vi "VI Tree.vi"   [LabVIEW 2020, in "Rohde&Schwarz CMXP GPRF.lvlib"]
doc: "This is the instrument driver for the R&S CMXP Radiocommunication Analyzer GPRF.\n\nThe VI Tree displays all the user-callable VIs of the instrument driver in an organized \ntable.\n\nFor detailed driver information including modification history, refer to the <B>rscmxpgprf.chm </B> file."
uses:
  <instrlib>/Rohde&Schwarz CMXP GPRF/Rohde&Schwarz CMXP GPRF.lvlib
panel:
  # "rsCmxpGprf"
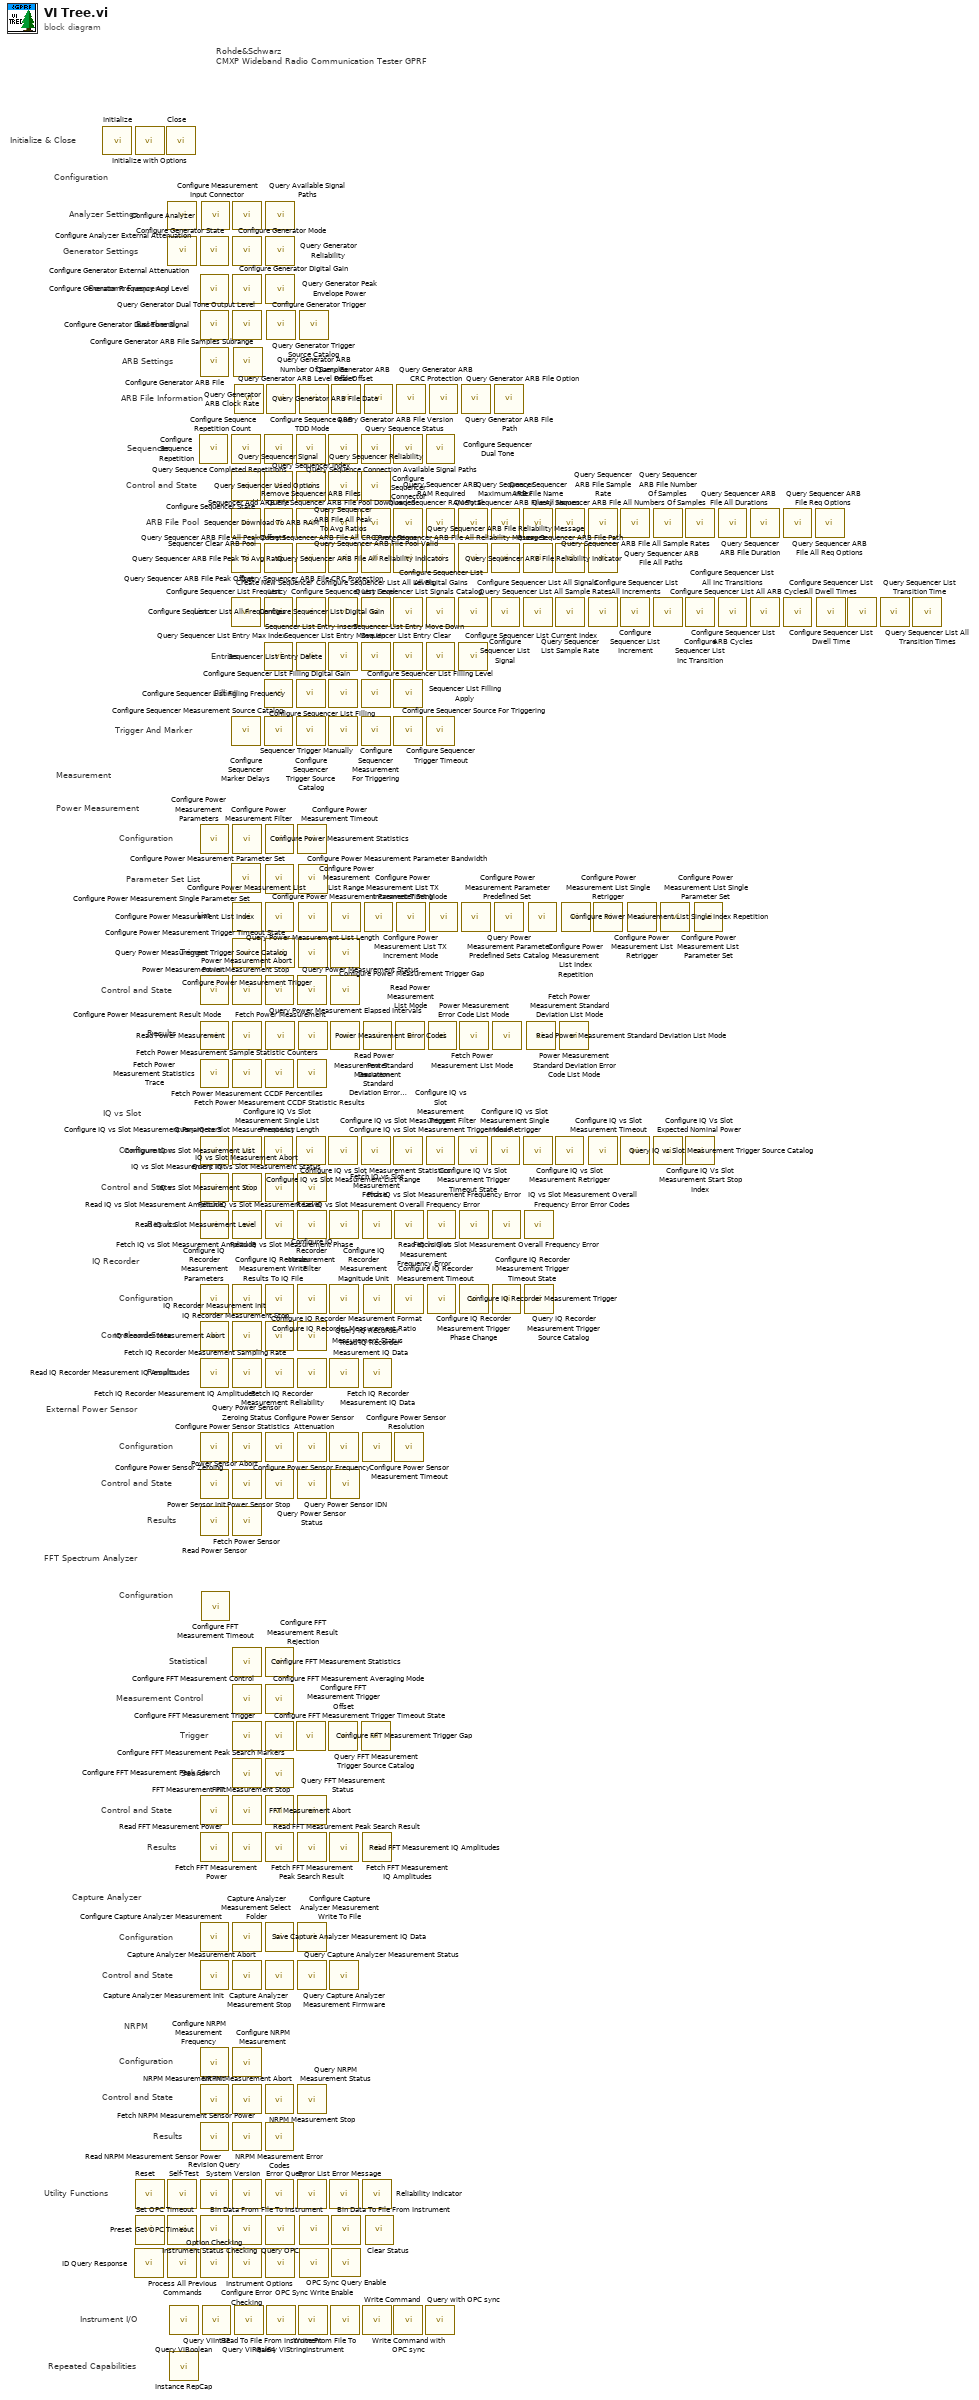
[diagram p0: block diagram]
diagram:
  # "Repeated Capabilities"
  # "Results"
  # "Control and State"
  # "Configuration"
  # "NRPM"
  # "Control and State"
  # "Configuration"
  # "Capture Analyzer"
  # "Trigger And Marker"
  # "Filling"
  # "Entries"
  # "List"
  # "ARB File Pool"
  # "Control and State"
  # "Sequencer"
  # "Parameter Set List"
  # "Rohde&Schwarz\nCMXP Wideband Radio Communication Tester GPRF"
  # "Instrument I/O"
  # "Utility Functions"
  # "Results"
  # "Control and State"
  # "Search"
  # "Trigger"
  # "Measurement Control"
  # "Statistical"
  # "Configuration"
  # "FFT Spectrum Analyzer"
  # "Results"
  # "Control and State"
  # "Configuration"
  # "External Power Sensor"
  # "Results"
  # "Control and State"
  # "Configuration"
  # "IQ Recorder"
  # "Results"
  # "Control and State"
  # "Configuration"
  # "IQ vs Slot"
  # "Results"
  # "Control and State"
  # "Trigger"
  # "List"
  # "Configuration"
  # "Power Measurement"
  # "Measurement"
  # "ARB File Information"
  # "ARB Settings"
  # "Baseband"
  # "Constant Frequency"
  # "Generator Settings"
  # "Analyzer Settings"
  # "Configuration"
  # "Initialize & Close"
  n1 = call <instrlib>:"Initialize.vi"() -> ()  [unwired: 10 in, 2 out]
  n2 = call <instrlib>:"ID Query Response.vi"() -> ()  [unwired: 9 in, 3 out]
  n3 = call <instrlib>:"Initialize with Options.vi"() -> ()  [unwired: 10 in, 2 out]
  n4 = call <instrlib>:"Reset.vi"() -> ()  [unwired: 10 in, 2 out]
  n5 = call <instrlib>:"Preset.vi"() -> ()  [unwired: 10 in, 2 out]
  n6 = call <instrlib>:"Close.vi"() -> ()  [unwired: 11 in, 1 out]
  n7 = call <instrlib>:"Configure Analyzer External Attenuation.vi"() -> ()  [unwired: 10 in, 2 out]
  n8 = call <instrlib>:"Configure Generator External Attenuation.vi"() -> ()  [unwired: 10 in, 2 out]
  n9 = call <instrlib>:"Self-Test.vi"() -> ()  [unwired: 8 in, 4 out]
  n10 = call <instrlib>:"Set OPC Timeout.vi"() -> ()  [unwired: 10 in, 2 out]
  n11 = call <instrlib>:"Process All Previous Commands.vi"() -> ()  [unwired: 10 in, 2 out]
  n12 = call <instrlib>:"Query ViBoolean.vi"() -> ()  [unwired: 9 in, 3 out]
  n13 = call <instrlib>:"Instance RepCap.vi"() -> ()  [unwired: 1 in, 1 out]
  n14 = call <instrlib>:"Configure Sequence Repetition.vi"() -> ()  [unwired: 10 in, 2 out]
  n15 = call <instrlib>:"Configure Generator State.vi"() -> ()  [unwired: 10 in, 2 out]
  n16 = call <instrlib>:"Configure Generator Frequency And Level.vi"() -> ()  [unwired: 10 in, 2 out]
  n17 = call <instrlib>:"Configure Generator Dual Tone Signal.vi"() -> ()  [unwired: 10 in, 2 out]
  n18 = call <instrlib>:"Configure Generator ARB File.vi"() -> ()  [unwired: 10 in, 2 out]
  n19 = call <instrlib>:"Configure Power Measurement Parameters.vi"() -> ()  [unwired: 10 in, 2 out]
  n20 = call <instrlib>:"Power Measurement Init.vi"() -> ()  [unwired: 10 in, 2 out]
  n21 = call <instrlib>:"Configure Power Measurement Result Mode.vi"() -> ()  [unwired: 10 in, 2 out]
  n22 = call <instrlib>:"Fetch Power Measurement Statistics Trace.vi"() -> ()  [unwired: 8 in, 4 out]
  n23 = call <instrlib>:"Configure IQ vs Slot Measurement Parameters.vi"() -> ()  [unwired: 10 in, 2 out]
  n24 = call <instrlib>:"IQ vs Slot Measurement Init.vi"() -> ()  [unwired: 10 in, 2 out]
  n25 = call <instrlib>:"Read IQ vs Slot Measurement Amplitude.vi"() -> ()  [unwired: 8 in, 4 out]
  n26 = call <instrlib>:"Configure IQ Recorder Measurement Parameters.vi"() -> ()  [unwired: 10 in, 2 out]
  n27 = call <instrlib>:"IQ Recorder Measurement Init.vi"() -> ()  [unwired: 10 in, 2 out]
  n28 = call <instrlib>:"Read IQ Recorder Measurement IQ Amplitudes.vi"() -> ()  [unwired: 7 in, 5 out]
  n29 = call <instrlib>:"Configure Power Sensor Zeroing.vi"() -> ()  [unwired: 10 in, 2 out]
  n30 = call <instrlib>:"Power Sensor Init.vi"() -> ()  [unwired: 10 in, 2 out]
  n31 = call <instrlib>:"Read Power Sensor.vi"() -> ()  [unwired: 7 in, 5 out]
  n32 = call <instrlib>:"FFT Measurement Init.vi"() -> ()  [unwired: 10 in, 2 out]
  n33 = call <instrlib>:"Read FFT Measurement Power.vi"() -> ()  [unwired: 8 in, 4 out]
  n34 = call <instrlib>:"Configure Capture Analyzer Measurement.vi"() -> ()  [unwired: 10 in, 2 out]
  n35 = call <instrlib>:"Capture Analyzer Measurement Init.vi"() -> ()  [unwired: 10 in, 2 out]
  n36 = call <instrlib>:"Configure NRPM Measurement Frequency.vi"() -> ()  [unwired: 10 in, 2 out]
  n37 = call <instrlib>:"NRPM Measurement Init.vi"() -> ()  [unwired: 10 in, 2 out]
  n38 = call <instrlib>:"Read NRPM Measurement Sensor Power.vi"() -> ()  [unwired: 8 in, 4 out]
  n39 = call <instrlib>:"Revision Query.vi"() -> ()  [unwired: 8 in, 4 out]
  n40 = call <instrlib>:"Get OPC Timeout.vi"() -> ()  [unwired: 9 in, 3 out]
  n41 = call <instrlib>:"Option Checking.vi"() -> ()  [unwired: 10 in, 2 out]
  n42 = call <instrlib>:"Configure Analyzer.vi"() -> ()  [unwired: 10 in, 2 out]
  n43 = call <instrlib>:"Configure FFT Measurement Timeout.vi"() -> ()  [unwired: 10 in, 2 out]
  n44 = call <instrlib>:"Query ViInt32.vi"() -> ()  [unwired: 9 in, 3 out]
  n45 = call <instrlib>:"Configure Sequence Repetition Count.vi"() -> ()  [unwired: 10 in, 2 out]
  n46 = call <instrlib>:"Configure Sequencer State.vi"() -> ()  [unwired: 10 in, 2 out]
  n47 = call <instrlib>:"Sequencer Clear ARB Pool.vi"() -> ()  [unwired: 10 in, 2 out]
  n48 = call <instrlib>:"Query Sequencer ARB File Peak Offset.vi"() -> ()  [unwired: 9 in, 3 out]
  n49 = call <instrlib>:"Create New Sequencer List.vi"() -> ()  [unwired: 10 in, 2 out]
  n50 = call <instrlib>:"Configure Sequencer Marker Delays.vi"() -> ()  [unwired: 10 in, 2 out]
  n51 = call <instrlib>:"Configure Power Measurement Single Parameter Set.vi"() -> ()  [unwired: 14 in, 2 out]
  n52 = call <instrlib>:"Configure Measurement Input Connector.vi"() -> ()  [unwired: 10 in, 2 out]
  n53 = call <instrlib>:"Configure Generator Mode.vi"() -> ()  [unwired: 10 in, 2 out]
  n54 = call <instrlib>:"Configure Generator Digital Gain.vi"() -> ()  [unwired: 10 in, 2 out]
  n55 = call <instrlib>:"Query Generator Dual Tone Output Level.vi"() -> ()  [unwired: 9 in, 3 out]
  n56 = call <instrlib>:"Configure Power Measurement Statistics.vi"() -> ()  [unwired: 10 in, 2 out]
  n57 = call <instrlib>:"Configure Power Measurement List.vi"() -> ()  [unwired: 10 in, 2 out]
  n58 = call <instrlib>:"Configure Power Measurement Trigger.vi"() -> ()  [unwired: 14 in, 2 out]
  n59 = call <instrlib>:"Power Measurement Abort.vi"() -> ()  [unwired: 10 in, 2 out]
  n60 = call <instrlib>:"Read Power Measurement.vi"() -> ()  [unwired: 8 in, 4 out]
  n61 = call <instrlib>:"Fetch Power Measurement CCDF Percentiles.vi"() -> ()  [unwired: 8 in, 4 out]
  n62 = call <instrlib>:"Configure IQ Vs Slot Measurement Single List Frequency.vi"() -> ()  [unwired: 10 in, 2 out]
  n63 = call <instrlib>:"IQ vs Slot Measurement Abort.vi"() -> ()  [unwired: 10 in, 2 out]
  n64 = call <instrlib>:"Fetch IQ vs Slot Measurement Amplitude.vi"() -> ()  [unwired: 8 in, 4 out]
  n65 = call <instrlib>:"Configure IQ Recorder Measurement Write Results To IQ File.vi"() -> ()  [unwired: 10 in, 2 out]
  n66 = call <instrlib>:"IQ Recorder Measurement Abort.vi"() -> ()  [unwired: 10 in, 2 out]
  n67 = call <instrlib>:"Fetch IQ Recorder Measurement IQ Amplitudes.vi"() -> ()  [unwired: 7 in, 5 out]
  n68 = call <instrlib>:"Query Power Sensor Zeroing Status.vi"() -> ()  [unwired: 8 in, 4 out]
  n69 = call <instrlib>:"Power Sensor Abort.vi"() -> ()  [unwired: 10 in, 2 out]
  n70 = call <instrlib>:"Fetch Power Sensor.vi"() -> ()  [unwired: 7 in, 5 out]
  n71 = call <instrlib>:"Configure FFT Measurement Statistics.vi"() -> ()  [unwired: 10 in, 2 out]
  n72 = call <instrlib>:"Configure FFT Measurement Control.vi"() -> ()  [unwired: 10 in, 2 out]
  n73 = call <instrlib>:"Configure FFT Measurement Trigger.vi"() -> ()  [unwired: 10 in, 2 out]
  n74 = call <instrlib>:"Configure FFT Measurement Peak Search.vi"() -> ()  [unwired: 10 in, 2 out]
  n75 = call <instrlib>:"FFT Measurement Abort.vi"() -> ()  [unwired: 10 in, 2 out]
  n76 = call <instrlib>:"Fetch FFT Measurement Power.vi"() -> ()  [unwired: 8 in, 4 out]
  n77 = call <instrlib>:"Save Capture Analyzer Measurement IQ Data.vi"() -> ()  [unwired: 10 in, 2 out]
  n78 = call <instrlib>:"Capture Analyzer Measurement Abort.vi"() -> ()  [unwired: 10 in, 2 out]
  n79 = call <instrlib>:"Configure NRPM Measurement.vi"() -> ()  [unwired: 10 in, 2 out]
  n80 = call <instrlib>:"NRPM Measurement Abort.vi"() -> ()  [unwired: 10 in, 2 out]
  n81 = call <instrlib>:"Fetch NRPM Measurement Sensor Power.vi"() -> ()  [unwired: 8 in, 4 out]
  n82 = call <instrlib>:"System Version.vi"() -> ()  [unwired: 9 in, 3 out]
  n83 = call <instrlib>:"Instrument Status Checking.vi"() -> ()  [unwired: 10 in, 2 out]
  n84 = call <instrlib>:"Configure Error Checking.vi"() -> ()  [unwired: 10 in, 2 out]
  n85 = call <instrlib>:"Configure Generator ARB File Samples Subrange.vi"() -> ()  [unwired: 10 in, 2 out]
  n86 = call <instrlib>:"Query Generator ARB File Date.vi"() -> ()  [unwired: 9 in, 3 out]
  n87 = call <instrlib>:"Query ViReal64.vi"() -> ()  [unwired: 9 in, 3 out]
  n88 = call <instrlib>:"Query Sequence Completed Repetitions.vi"() -> ()  [unwired: 9 in, 3 out]
  n89 = call <instrlib>:"Query Sequencer Signal.vi"() -> ()  [unwired: 9 in, 3 out]
  n90 = call <instrlib>:"Sequencer Add ARB File.vi"() -> ()  [unwired: 10 in, 2 out]
  n91 = call <instrlib>:"Query Sequencer ARB File All Peak Offsets.vi"() -> ()  [unwired: 9 in, 3 out]
  n92 = call <instrlib>:"Configure Sequencer List Frequency.vi"() -> ()  [unwired: 10 in, 2 out]
  n93 = call <instrlib>:"Query Sequencer List Entry Max Index.vi"() -> ()  [unwired: 9 in, 3 out]
  n94 = call <instrlib>:"Configure Sequencer List Filling.vi"() -> ()  [unwired: 10 in, 2 out]
  n95 = call <instrlib>:"Configure Sequencer Measurement Source Catalog.vi"() -> ()  [unwired: 9 in, 3 out]
  n96 = call <instrlib>:"Configure IQ vs Slot Measurement List.vi"() -> ()  [unwired: 10 in, 2 out]
  n97 = call <instrlib>:"Configure Power Measurement Filter.vi"() -> ()  [unwired: 10 in, 2 out]
  n98 = call <instrlib>:"Configure Power Measurement Parameter Set.vi"() -> ()  [unwired: 10 in, 2 out]
  n99 = call <instrlib>:"Configure Power Measurement List Index.vi"() -> ()  [unwired: 10 in, 2 out]
  n100 = call <instrlib>:"Power Measurement Stop.vi"() -> ()  [unwired: 10 in, 2 out]
  n101 = call <instrlib>:"Fetch Power Measurement CCDF Statistic Results.vi"() -> ()  [unwired: 5 in, 7 out]
  n102 = call <instrlib>:"IQ vs Slot Measurement Stop.vi"() -> ()  [unwired: 10 in, 2 out]
  n103 = call <instrlib>:"Read IQ vs Slot Measurement Level.vi"() -> ()  [unwired: 8 in, 4 out]
  n104 = call <instrlib>:"Configure IQ Recorder Measurement Format.vi"() -> ()  [unwired: 10 in, 2 out]
  n105 = call <instrlib>:"IQ Recorder Measurement Stop.vi"() -> ()  [unwired: 10 in, 2 out]
  n106 = call <instrlib>:"Fetch IQ Recorder Measurement Sampling Rate.vi"() -> ()  [unwired: 9 in, 3 out]
  n107 = call <instrlib>:"Configure Power Sensor Statistics.vi"() -> ()  [unwired: 10 in, 2 out]
  n108 = call <instrlib>:"Power Sensor Stop.vi"() -> ()  [unwired: 10 in, 2 out]
  n109 = call <instrlib>:"Configure FFT Measurement Result Rejection.vi"() -> ()  [unwired: 10 in, 2 out]
  n110 = call <instrlib>:"Configure FFT Measurement Averaging Mode.vi"() -> ()  [unwired: 10 in, 2 out]
  n111 = call <instrlib>:"Configure FFT Measurement Trigger Timeout State.vi"() -> ()  [unwired: 10 in, 2 out]
  n112 = call <instrlib>:"Configure FFT Measurement Peak Search Markers.vi"() -> ()  [unwired: 10 in, 2 out]
  n113 = call <instrlib>:"FFT Measurement Stop.vi"() -> ()  [unwired: 10 in, 2 out]
  n114 = call <instrlib>:"Read FFT Measurement Peak Search Result.vi"() -> ()  [unwired: 7 in, 5 out]
  n115 = call <instrlib>:"Capture Analyzer Measurement Select Folder.vi"() -> ()  [unwired: 10 in, 2 out]
  n116 = call <instrlib>:"Capture Analyzer Measurement Stop.vi"() -> ()  [unwired: 10 in, 2 out]
  n117 = call <instrlib>:"NRPM Measurement Stop.vi"() -> ()  [unwired: 10 in, 2 out]
  n118 = call <instrlib>:"NRPM Measurement Error Codes.vi"() -> ()  [unwired: 8 in, 4 out]
  n119 = call <instrlib>:"Error Query.vi"() -> ()  [unwired: 8 in, 4 out]
  n120 = call <instrlib>:"Query Available Signal Paths.vi"() -> ()  [unwired: 9 in, 3 out]
  n121 = call <instrlib>:"Query Generator Reliability.vi"() -> ()  [unwired: 7 in, 5 out]
  n122 = call <instrlib>:"Query Generator Peak Envelope Power.vi"() -> ()  [unwired: 9 in, 3 out]
  n123 = call <instrlib>:"Configure Power Measurement Trigger Timeout State.vi"() -> ()  [unwired: 10 in, 2 out]
  n124 = call <instrlib>:"Fetch Power Measurement.vi"() -> ()  [unwired: 8 in, 4 out]
  n125 = call <instrlib>:"Query OPC.vi"() -> ()  [unwired: 9 in, 3 out]
  n126 = call <instrlib>:"Instrument Options.vi"() -> ()  [unwired: 9 in, 3 out]
  n127 = call <instrlib>:"Configure Generator Trigger.vi"() -> ()  [unwired: 10 in, 2 out]
  n128 = call <instrlib>:"Query Generator ARB Clock Rate.vi"() -> ()  [unwired: 9 in, 3 out]
  n129 = call <instrlib>:"Query ViString.vi"() -> ()  [unwired: 9 in, 3 out]
  n130 = call <instrlib>:"Query Sequence Connection Available Signal Paths.vi"() -> ()  [unwired: 9 in, 3 out]
  n131 = call <instrlib>:"Query Sequencer Index.vi"() -> ()  [unwired: 9 in, 3 out]
  n132 = call <instrlib>:"Remove Sequencer ARB Files.vi"() -> ()  [unwired: 10 in, 2 out]
  n133 = call <instrlib>:"Query Sequencer ARB File Peak To Avg Ratio.vi"() -> ()  [unwired: 9 in, 3 out]
  n134 = call <instrlib>:"Configure Sequencer List All Frequencies.vi"() -> ()  [unwired: 10 in, 2 out]
  n135 = call <instrlib>:"Sequencer List Entry Insert.vi"() -> ()  [unwired: 10 in, 2 out]
  n136 = call <instrlib>:"Configure Sequencer List Filling Frequency.vi"() -> ()  [unwired: 10 in, 2 out]
  n137 = call <instrlib>:"Configure Sequencer Trigger Source Catalog.vi"() -> ()  [unwired: 9 in, 3 out]
  n138 = call <instrlib>:"Query IQ vs Slot Measurement List Length.vi"() -> ()  [unwired: 9 in, 3 out]
  n139 = call <instrlib>:"Configure FFT Measurement Trigger Gap.vi"() -> ()  [unwired: 10 in, 2 out]
  n140 = call <instrlib>:"Configure Power Measurement Timeout.vi"() -> ()  [unwired: 10 in, 2 out]
  n141 = call <instrlib>:"Query Power Measurement Status.vi"() -> ()  [unwired: 7 in, 5 out]
  n142 = call <instrlib>:"Fetch Power Measurement Sample Statistic Counters.vi"() -> ()  [unwired: 7 in, 5 out]
  n143 = call <instrlib>:"Query IQ vs Slot Measurement Status.vi"() -> ()  [unwired: 7 in, 5 out]
  n144 = call <instrlib>:"Fetch IQ vs Slot Measurement Level.vi"() -> ()  [unwired: 8 in, 4 out]
  n145 = call <instrlib>:"Configure IQ Recorder Measurement Filter.vi"() -> ()  [unwired: 10 in, 2 out]
  n146 = call <instrlib>:"Query IQ Recorder Measurement Status.vi"() -> ()  [unwired: 7 in, 5 out]
  n147 = call <instrlib>:"Fetch IQ Recorder Measurement Reliability.vi"() -> ()  [unwired: 9 in, 3 out]
  n148 = call <instrlib>:"Configure Power Sensor Frequency.vi"() -> ()  [unwired: 10 in, 2 out]
  n149 = call <instrlib>:"Query Power Sensor Status.vi"() -> ()  [unwired: 7 in, 5 out]
  n150 = call <instrlib>:"Query FFT Measurement Status.vi"() -> ()  [unwired: 7 in, 5 out]
  n151 = call <instrlib>:"Fetch FFT Measurement Peak Search Result.vi"() -> ()  [unwired: 7 in, 5 out]
  n152 = call <instrlib>:"Configure Capture Analyzer Measurement Write To File.vi"() -> ()  [unwired: 10 in, 2 out]
  n153 = call <instrlib>:"Query Capture Analyzer Measurement Status.vi"() -> ()  [unwired: 7 in, 5 out]
  n154 = call <instrlib>:"Query NRPM Measurement Status.vi"() -> ()  [unwired: 7 in, 5 out]
  n155 = call <instrlib>:"Error List.vi"() -> ()  [unwired: 9 in, 3 out]
  n156 = call <instrlib>:"Configure Power Measurement Parameter Bandwidth.vi"() -> ()  [unwired: 10 in, 2 out]
  n157 = call <instrlib>:"Query Power Measurement List Length.vi"() -> ()  [unwired: 9 in, 3 out]
  n158 = call <instrlib>:"Query Power Measurement Trigger Source Catalog.vi"() -> ()  [unwired: 9 in, 3 out]
  n159 = call <instrlib>:"Power Measurement Error Codes.vi"() -> ()  [unwired: 8 in, 4 out]
  n160 = call <instrlib>:"Read To File From Instrument.vi"() -> ()  [unwired: 10 in, 2 out]
  n161 = call <instrlib>:"Query Generator Trigger Source Catalog.vi"() -> ()  [unwired: 9 in, 3 out]
  n162 = call <instrlib>:"Query Generator ARB Number Of Samples.vi"() -> ()  [unwired: 9 in, 3 out]
  n163 = call <instrlib>:"Bin Data From File To Instrument.vi"() -> ()  [unwired: 10 in, 2 out]
  n164 = call <instrlib>:"OPC Sync Write Enable.vi"() -> ()  [unwired: 10 in, 2 out]
  n165 = call <instrlib>:"Configure Sequence ARB TDD Mode.vi"() -> ()  [unwired: 10 in, 2 out]
  n166 = call <instrlib>:"Query Sequencer Used Options.vi"() -> ()  [unwired: 9 in, 3 out]
  n167 = call <instrlib>:"Sequencer Download To ARB RAM.vi"() -> ()  [unwired: 10 in, 2 out]
  n168 = call <instrlib>:"Query Sequencer ARB File All Peak To Avg Ratios.vi"() -> ()  [unwired: 9 in, 3 out]
  n169 = call <instrlib>:"Configure Sequencer List Level.vi"() -> ()  [unwired: 10 in, 2 out]
  n170 = call <instrlib>:"Sequencer List Entry Delete.vi"() -> ()  [unwired: 10 in, 2 out]
  n171 = call <instrlib>:"Configure Sequencer List Filling Digital Gain.vi"() -> ()  [unwired: 10 in, 2 out]
  n172 = call <instrlib>:"Sequencer Trigger Manually.vi"() -> ()  [unwired: 10 in, 2 out]
  n173 = call <instrlib>:"Configure IQ vs Slot Measurement List Range.vi"() -> ()  [unwired: 10 in, 2 out]
  n174 = call <instrlib>:"Configure FFT Measurement Trigger Offset.vi"() -> ()  [unwired: 10 in, 2 out]
  n175 = call <instrlib>:"Read IQ vs Slot Measurement Phase.vi"() -> ()  [unwired: 8 in, 4 out]
  n176 = call <instrlib>:"Configure IQ Recorder Measurement Ratio.vi"() -> ()  [unwired: 10 in, 2 out]
  n177 = call <instrlib>:"Read IQ Recorder Measurement IQ Data.vi"() -> ()  [unwired: 8 in, 4 out]
  n178 = call <instrlib>:"Configure Power Sensor Attenuation.vi"() -> ()  [unwired: 10 in, 2 out]
  n179 = call <instrlib>:"Read FFT Measurement IQ Amplitudes.vi"() -> ()  [unwired: 8 in, 4 out]
  n180 = call <instrlib>:"Query Capture Analyzer Measurement Firmware.vi"() -> ()  [unwired: 9 in, 3 out]
  n181 = call <instrlib>:"Error Message.vi"() -> ()  [unwired: 7 in, 5 out]
  n182 = call <instrlib>:"Configure Power Measurement Trigger Gap.vi"() -> ()  [unwired: 10 in, 2 out]
  n183 = call <instrlib>:"Query Power Measurement Elapsed Intervals.vi"() -> ()  [unwired: 9 in, 3 out]
  n184 = call <instrlib>:"Read Power Measurement Standard Deviation.vi"() -> ()  [unwired: 8 in, 4 out]
  n185 = call <instrlib>:"Query Power Sensor IDN.vi"() -> ()  [unwired: 9 in, 3 out]
  n186 = call <instrlib>:"Write From File To Instrument.vi"() -> ()  [unwired: 10 in, 2 out]
  n187 = call <instrlib>:"Query Generator ARB Level Offset.vi"() -> ()  [unwired: 9 in, 3 out]
  n188 = call <instrlib>:"Configure Power Measurement List Range.vi"() -> ()  [unwired: 10 in, 2 out]
  n189 = call <instrlib>:"Bin Data To File From Instrument.vi"() -> ()  [unwired: 10 in, 2 out]
  n190 = call <instrlib>:"OPC Sync Query Enable.vi"() -> ()  [unwired: 10 in, 2 out]
  n191 = call <instrlib>:"Query Sequence Status.vi"() -> ()  [unwired: 11 in, 5 out]
  n192 = call <instrlib>:"Query Sequencer Reliability.vi"() -> ()  [unwired: 7 in, 5 out]
  n193 = call <instrlib>:"Query Sequencer ARB File Pool Valid.vi"() -> ()  [unwired: 9 in, 3 out]
  n194 = call <instrlib>:"Query Sequencer ARB File CRC Protection.vi"() -> ()  [unwired: 9 in, 3 out]
  n195 = call <instrlib>:"Configure Sequencer List All Levels.vi"() -> ()  [unwired: 10 in, 2 out]
  n196 = call <instrlib>:"Sequencer List Entry Move Up.vi"() -> ()  [unwired: 10 in, 2 out]
  n197 = call <instrlib>:"Configure Sequencer List Filling Level.vi"() -> ()  [unwired: 10 in, 2 out]
  n198 = call <instrlib>:"Configure Sequencer Measurement For Triggering.vi"() -> ()  [unwired: 10 in, 2 out]
  n199 = call <instrlib>:"Configure IQ vs Slot Measurement Statistics.vi"() -> ()  [unwired: 10 in, 2 out]
  n200 = call <instrlib>:"Query FFT Measurement Trigger Source Catalog.vi"() -> ()  [unwired: 9 in, 3 out]
  n201 = call <instrlib>:"Fetch IQ vs Slot Measurement Phase.vi"() -> ()  [unwired: 8 in, 4 out]
  n202 = call <instrlib>:"Configure Power Sensor Resolution.vi"() -> ()  [unwired: 10 in, 2 out]
  n203 = call <instrlib>:"Fetch FFT Measurement IQ Amplitudes.vi"() -> ()  [unwired: 8 in, 4 out]
  n204 = call <instrlib>:"Reliability Indicator.vi"() -> ()  [unwired: 9 in, 3 out]
  n205 = call <instrlib>:"Write Command.vi"() -> ()  [unwired: 10 in, 2 out]
  n206 = call <instrlib>:"Power Measurement Standard Deviation Error Codes.vi"() -> ()  [unwired: 8 in, 4 out]
  n207 = call <instrlib>:"Configure IQ Recorder Measurement Magnitude Unit.vi"() -> ()  [unwired: 10 in, 2 out]
  n208 = call <instrlib>:"Fetch IQ Recorder Measurement IQ Data.vi"() -> ()  [unwired: 8 in, 4 out]
  n209 = call <instrlib>:"Query Generator ARB Peak Offset.vi"() -> ()  [unwired: 9 in, 3 out]
  n210 = call <instrlib>:"Configure Power Measurement List TX Increment Timing.vi"() -> ()  [unwired: 10 in, 2 out]
  n211 = call <instrlib>:"Clear Status.vi"() -> ()  [unwired: 10 in, 2 out]
  n212 = call <instrlib>:"Configure Sequencer Connector.vi"() -> ()  [unwired: 10 in, 2 out]
  n213 = call <instrlib>:"Query Sequencer ARB File Pool Downloaded.vi"() -> ()  [unwired: 9 in, 3 out]
  n214 = call <instrlib>:"Query Sequencer ARB File All CRC Protections.vi"() -> ()  [unwired: 9 in, 3 out]
  n215 = call <instrlib>:"Configure Sequencer List Digital Gain.vi"() -> ()  [unwired: 10 in, 2 out]
  n216 = call <instrlib>:"Sequencer List Entry Move Down.vi"() -> ()  [unwired: 10 in, 2 out]
  n217 = call <instrlib>:"Sequencer List Filling Apply.vi"() -> ()  [unwired: 10 in, 2 out]
  n218 = call <instrlib>:"Configure Sequencer Source For Triggering.vi"() -> ()  [unwired: 10 in, 2 out]
  n219 = call <instrlib>:"Configure IQ vs Slot Measurement Filter.vi"() -> ()  [unwired: 10 in, 2 out]
  n220 = call <instrlib>:"Write Command with OPC sync.vi"() -> ()  [unwired: 10 in, 2 out]
  n221 = call <instrlib>:"Read IQ vs Slot Measurement Frequency Error.vi"() -> ()  [unwired: 8 in, 4 out]
  n222 = call <instrlib>:"Configure IQ Recorder Measurement Timeout.vi"() -> ()  [unwired: 10 in, 2 out]
  n223 = call <instrlib>:"Configure Power Sensor Measurement Timeout.vi"() -> ()  [unwired: 10 in, 2 out]
  n224 = call <instrlib>:"Read Power Measurement List Mode.vi"() -> ()  [unwired: 8 in, 4 out]
  n225 = call <instrlib>:"Query Generator ARB CRC Protection.vi"() -> ()  [unwired: 9 in, 3 out]
  n226 = call <instrlib>:"Configure Power Measurement List TX Increment Mode.vi"() -> ()  [unwired: 10 in, 2 out]
  n227 = call <instrlib>:"Query with OPC sync.vi"() -> ()  [unwired: 9 in, 3 out]
  n228 = call <instrlib>:"Configure Sequencer Dual Tone.vi"() -> ()  [unwired: 10 in, 2 out]
  n229 = call <instrlib>:"Query Sequencer ARB RAM Required.vi"() -> ()  [unwired: 9 in, 3 out]
  n230 = call <instrlib>:"Query Sequencer ARB File Reliability Indicator.vi"() -> ()  [unwired: 9 in, 3 out]
  n231 = call <instrlib>:"Configure Sequencer List All Digital Gains.vi"() -> ()  [unwired: 10 in, 2 out]
  n232 = call <instrlib>:"Sequencer List Entry Clear.vi"() -> ()  [unwired: 10 in, 2 out]
  n233 = call <instrlib>:"Configure Sequencer Trigger Timeout.vi"() -> ()  [unwired: 10 in, 2 out]
  n234 = call <instrlib>:"Configure IQ vs Slot Measurement Trigger.vi"() -> ()  [unwired: 14 in, 2 out]
  n235 = call <instrlib>:"Fetch IQ vs Slot Measurement Frequency Error.vi"() -> ()  [unwired: 8 in, 4 out]
  n236 = call <instrlib>:"Configure IQ Recorder Measurement Trigger.vi"() -> ()  [unwired: 14 in, 2 out]
  n237 = call <instrlib>:"Fetch Power Measurement List Mode.vi"() -> ()  [unwired: 8 in, 4 out]
  n238 = call <instrlib>:"Query Generator ARB File Version.vi"() -> ()  [unwired: 9 in, 3 out]
  n239 = call <instrlib>:"Configure Power Measurement Parameter Set Mode.vi"() -> ()  [unwired: 10 in, 2 out]
  n240 = call <instrlib>:"Query Sequencer RAM Total.vi"() -> ()  [unwired: 9 in, 3 out]
  n241 = call <instrlib>:"Query Sequencer ARB File All Reliability Indicators.vi"() -> ()  [unwired: 9 in, 3 out]
  n242 = call <instrlib>:"Query Sequencer List Signals Catalog.vi"() -> ()  [unwired: 9 in, 3 out]
  n243 = call <instrlib>:"Configure Sequencer List Current Index.vi"() -> ()  [unwired: 10 in, 2 out]
  n244 = call <instrlib>:"Configure IQ Vs Slot Measurement Trigger Timeout State.vi"() -> ()  [unwired: 10 in, 2 out]
  n245 = call <instrlib>:"Power Measurement Error Code List Mode.vi"() -> ()  [unwired: 9 in, 3 out]
  n246 = call <instrlib>:"Read IQ vs Slot Measurement Overall Frequency Error.vi"() -> ()  [unwired: 8 in, 4 out]
  n247 = call <instrlib>:"Configure IQ Recorder Measurement Trigger Phase Change.vi"() -> ()  [unwired: 10 in, 2 out]
  n248 = call <instrlib>:"Query Generator ARB File Option.vi"() -> ()  [unwired: 9 in, 3 out]
  n249 = call <instrlib>:"Configure Power Measurement Parameter Predefined Set.vi"() -> ()  [unwired: 10 in, 2 out]
  n250 = call <instrlib>:"Query Sequencer Maximum Index.vi"() -> ()  [unwired: 9 in, 3 out]
  n251 = call <instrlib>:"Query Sequencer ARB File Reliability Message.vi"() -> ()  [unwired: 9 in, 3 out]
  n252 = call <instrlib>:"Configure Sequencer List Signal.vi"() -> ()  [unwired: 10 in, 2 out]
  n253 = call <instrlib>:"Configure IQ vs Slot Measurement Trigger Mode.vi"() -> ()  [unwired: 10 in, 2 out]
  n254 = call <instrlib>:"Fetch IQ vs Slot Measurement Overall Frequency Error.vi"() -> ()  [unwired: 8 in, 4 out]
  n255 = call <instrlib>:"Configure IQ Recorder Measurement Trigger Timeout State.vi"() -> ()  [unwired: 10 in, 2 out]
  n256 = call <instrlib>:"Read Power Measurement Standard Deviation List Mode.vi"() -> ()  [unwired: 8 in, 4 out]
  n257 = call <instrlib>:"Query Generator ARB File Path.vi"() -> ()  [unwired: 9 in, 3 out]
  n258 = call <instrlib>:"Query Power Measurement Parameter Predefined Sets Catalog.vi"() -> ()  [unwired: 9 in, 3 out]
  n259 = call <instrlib>:"Query Sequencer ARB File Name.vi"() -> ()  [unwired: 9 in, 3 out]
  n260 = call <instrlib>:"Query Sequencer ARB File All Reliability Messages.vi"() -> ()  [unwired: 9 in, 3 out]
  n261 = call <instrlib>:"Configure Sequencer List All Signals.vi"() -> ()  [unwired: 10 in, 2 out]
  n262 = call <instrlib>:"Configure IQ vs Slot Measurement Single Index Retrigger.vi"() -> ()  [unwired: 10 in, 2 out]
  n263 = call <instrlib>:"IQ vs Slot Measurement Overall Frequency Error Error Codes.vi"() -> ()  [unwired: 8 in, 4 out]
  n264 = call <instrlib>:"Query IQ Recorder Measurement Trigger Source Catalog.vi"() -> ()  [unwired: 9 in, 3 out]
  n265 = call <instrlib>:"Fetch Power Measurement Standard Deviation List Mode.vi"() -> ()  [unwired: 8 in, 4 out]
  n266 = call <instrlib>:"Configure Power Measurement List Single Index Repetition.vi"() -> ()  [unwired: 10 in, 2 out]
  n267 = call <instrlib>:"Configure IQ vs Slot Measurement Retrigger.vi"() -> ()  [unwired: 10 in, 2 out]
  n268 = call <instrlib>:"Query Sequencer ARB File All Names.vi"() -> ()  [unwired: 9 in, 3 out]
  n269 = call <instrlib>:"Query Sequencer ARB File Path.vi"() -> ()  [unwired: 9 in, 3 out]
  n270 = call <instrlib>:"Query Sequencer List Sample Rate.vi"() -> ()  [unwired: 9 in, 3 out]
  n271 = call <instrlib>:"Power Measurement Standard Deviation Error Code List Mode.vi"() -> ()  [unwired: 9 in, 3 out]
  n272 = call <instrlib>:"Configure Power Measurement List Index Repetition.vi"() -> ()  [unwired: 10 in, 2 out]
  n273 = call <instrlib>:"Query Sequencer ARB File Sample Rate.vi"() -> ()  [unwired: 9 in, 3 out]
  n274 = call <instrlib>:"Query Sequencer ARB File All Paths.vi"() -> ()  [unwired: 9 in, 3 out]
  n275 = call <instrlib>:"Query Sequencer List All Sample Rates.vi"() -> ()  [unwired: 9 in, 3 out]
  n276 = call <instrlib>:"Query IQ vs Slot Measurement Trigger Source Catalog.vi"() -> ()  [unwired: 9 in, 3 out]
  n277 = call <instrlib>:"Configure Power Measurement List Single Retrigger.vi"() -> ()  [unwired: 10 in, 2 out]
  n278 = call <instrlib>:"Query Sequencer ARB File All Sample Rates.vi"() -> ()  [unwired: 9 in, 3 out]
  n279 = call <instrlib>:"Configure Sequencer List Increment.vi"() -> ()  [unwired: 10 in, 2 out]
  n280 = call <instrlib>:"Configure IQ vs Slot Measurement Timeout.vi"() -> ()  [unwired: 10 in, 2 out]
  n281 = call <instrlib>:"Configure Power Measurement List Retrigger.vi"() -> ()  [unwired: 10 in, 2 out]
  n282 = call <instrlib>:"Query Sequencer ARB File Number Of Samples.vi"() -> ()  [unwired: 9 in, 3 out]
  n283 = call <instrlib>:"Configure Sequencer List All Increments.vi"() -> ()  [unwired: 10 in, 2 out]
  n284 = call <instrlib>:"Configure IQ Vs Slot Expected Nominal Power.vi"() -> ()  [unwired: 10 in, 2 out]
  n285 = call <instrlib>:"Configure Power Measurement List Single Parameter Set.vi"() -> ()  [unwired: 10 in, 2 out]
  n286 = call <instrlib>:"Query Sequencer ARB File All Numbers Of Samples.vi"() -> ()  [unwired: 9 in, 3 out]
  n287 = call <instrlib>:"Configure Sequencer List Inc Transition.vi"() -> ()  [unwired: 10 in, 2 out]
  n288 = call <instrlib>:"Configure IQ Vs Slot Measurement Start Stop Index.vi"() -> ()  [unwired: 10 in, 2 out]
  n289 = call <instrlib>:"Configure Power Measurement List Parameter Set.vi"() -> ()  [unwired: 10 in, 2 out]
  n290 = call <instrlib>:"Query Sequencer ARB File Duration.vi"() -> ()  [unwired: 9 in, 3 out]
  n291 = call <instrlib>:"Configure Sequencer List All Inc Transitions.vi"() -> ()  [unwired: 10 in, 2 out]
  n292 = call <instrlib>:"Query Sequencer ARB File All Durations.vi"() -> ()  [unwired: 9 in, 3 out]
  n293 = call <instrlib>:"Configure Sequencer List ARB Cycles.vi"() -> ()  [unwired: 10 in, 2 out]
  n294 = call <instrlib>:"Query Sequencer ARB File Req Options.vi"() -> ()  [unwired: 9 in, 3 out]
  n295 = call <instrlib>:"Configure Sequencer List All ARB Cycles.vi"() -> ()  [unwired: 10 in, 2 out]
  n296 = call <instrlib>:"Query Sequencer ARB File All Req Options.vi"() -> ()  [unwired: 9 in, 3 out]
  n297 = call <instrlib>:"Configure Sequencer List Dwell Time.vi"() -> ()  [unwired: 10 in, 2 out]
  n298 = call <instrlib>:"Configure Sequencer List All Dwell Times.vi"() -> ()  [unwired: 10 in, 2 out]
  n299 = call <instrlib>:"Query Sequencer List Transition Time.vi"() -> ()  [unwired: 9 in, 3 out]
  n300 = call <instrlib>:"Query Sequencer List All Transition Times.vi"() -> ()  [unwired: 9 in, 3 out]
